vi "ma_sml_Peak Rough Search Indices (basic).vi"(0 "x":dbl[](array[numeric]) format="%.5e", 1 "threshold":dbl=-inf format="%.2f", 2 "FFT Size":i32=1024, 3 "Window Size":i32=1024, 4 "window":u16(ring) items=["Rectangle"=0, "Hanning"=1, "Hamming"=2, "Blackman-Harris"=3, "Exact Blackman"=4, "Blackman"=5, "Flat Top"=6, "4 Term B-Harris "=7, "7 Term B-Harris"=8, "Low Sidelobe"=9, "Blackman Nuttall"=11, "Triangle"=30, "Bartlett-Hanning"=31, "Bohman"=32, "Parzen"=33, "Welch"=34, "Kaiser"=60, "Dolph-Chebyshev"=61, "Gaussian"=62]) -> (5 "peak indice":i32[](array[numeric]))   [LabVIEW 2020, in "NI_MAPro.lvlib"]
uses:
  NI_MAPro.lvlib
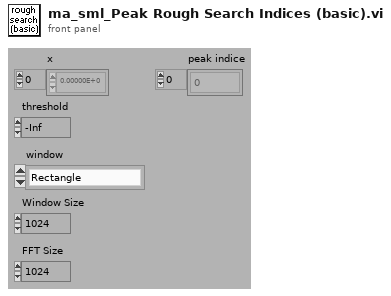
[diagram p1: front panel]
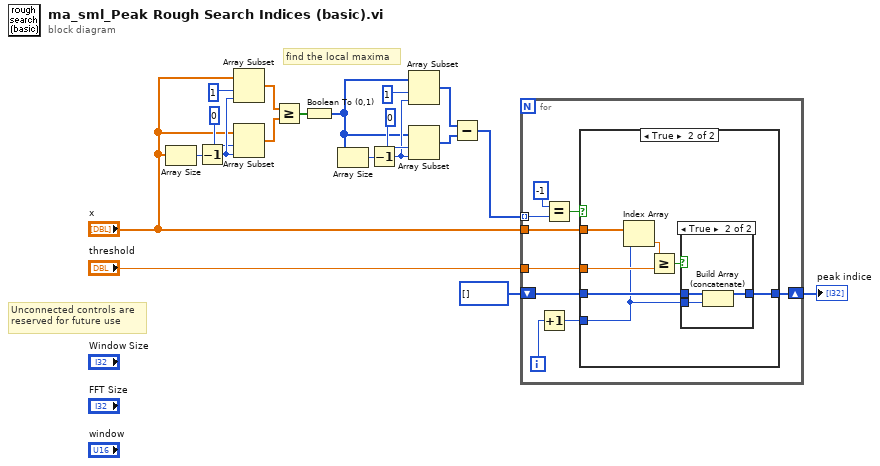
[diagram p0: block diagram]
diagram:
  # "Unconnected controls are\nreserved for future use"
  # "find the local maxima"
  n1 = Array Size(array="x") -> (size(s)=w18:i32)
  n2 = Decrement(x=w18) -> (x-1=w17:i32)
  n3 = Array Subset(array="x", index=1, length=w17) -> (w14:dbl[])
  n4 = Array Subset(array="x", index=0, length=w17) -> (w13:dbl[])
  n5 = Greater Or Equal?(x=w14, y=w13) -> (x >= y?=w12:bool[])
  n6 = Boolean To (0,1)(Boolean=w12) -> (0, 1=w7:i16[])
  n7 = Array Size(array=w7) -> (size(s)=w8:i32)
  n8 = Decrement(x=w8) -> (x-1=w9:i32)
  n9 = Array Subset(array=w7, index=1, length=w9) -> (w6:i16[])
  n10 = Array Subset(array=w7, index=0, length=w9) -> (w5:i16[])
  n11 = Subtract(x=w6, y=w5) -> (x-y=w2:i16[])
  n12 = for {
    shift-right: [w23] -> w3
    shift-left: i32[] [] -> [w24]
    tunnel: w2 -> [w22] mode=indexing
    tunnel: "x" -> [w26]
    tunnel: "threshold" -> [w25]
    i -> [w21]
    n13 = Increment(x=w21) -> (x+1=w20:i32)
    n14 = Equal?(x=i16 -1, y=w22) -> (x = y?=w27:bool)
    n15 = case shown="True" w27 {
      tunnel: w26 -> [_ w36]
      tunnel: w25 -> [_ w35]
      tunnel: w24 -> [w29 w34]
      tunnel: [w29 w33] -> w23
      tunnel: w20 -> [_ w32]
      frame False {
      }
      frame True {
        n16 = Index Array(array=w36, index=w32) -> (element=w31:dbl)
        n17 = Greater Or Equal?(x=w31, y=w35) -> (x >= y?=w30:bool)
        n18 = case shown="True" w30 {
          tunnel: w32 -> [_ w40]
          tunnel: w34 -> [w37 w39]
          tunnel: [w37 w38] -> w33
          frame False {
          }
          frame True {
            n19 = Build Array (concatenate)(w39, w40) -> (w38:i32[])
          }
        }
      }
    }
  }
  "peak indice" <- w3
